vi "Do.vi"(8 "error in":errorcluster, 10 "Actor in":refnum<class "Actor.lvclass">, 11 "Data MSG":refnum<class "Data MSG.lvclass">) -> (0 "error out":errorcluster, 2 "Actor out":refnum<class "Actor.lvclass">)   [LabVIEW 2014, in "Instrument Library.lvlib" / "Data MSG.lvclass"]
doc: "(<B>Filename</B>: Actor Framework.lvlib:Message.lvclass:Do.vi)\n\nDefines what a message does when it is received by an actor. Generally, a message instructs an actor to invoke one of its methods. By default, this method does nothing. A child class must override it to define behavior. Create a child class by using the Actor Framework Message Maker dialog box."
uses:
  Data MSG.lvclass
  <vilib>/ActorFramework/Actor/Actor.lvclass
  Instr Actor/Instr Actor.lvclass
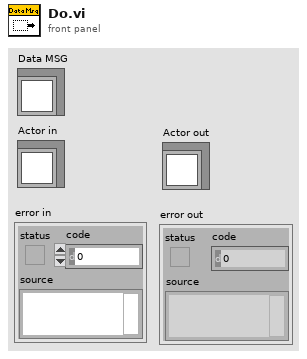
[diagram p1: front panel]
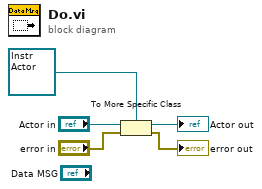
[diagram p0: block diagram]
diagram:
  n1 = To More Specific Class(target class=refnum<class "Instr Actor.lvclass"> refnum ("Instr Actor.lvclass"), reference="Actor in", error in="error in") -> (specific class reference=→"Actor out":refnum<class "Instr Actor.lvclass">, error out=→"error out":errorcluster)
